vi "LineCrossed.vi"() -> (1 "LineDir":bool, 3 "Onside":bool)   [LabVIEW 2013]
uses:
  Robot Global Data.vi
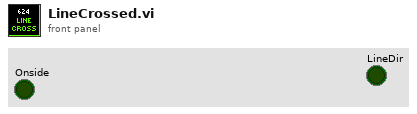
[diagram p1: front panel]
types:
  T1 = typedef "WPI_DriverStationAllianceInfo.ctl" = enum16{"Red", "Blue", "Invalid"}
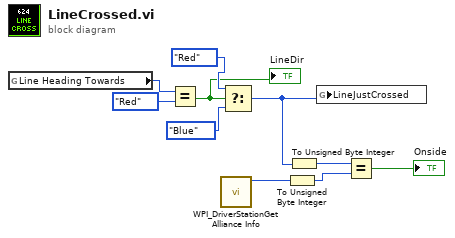
[diagram p0: block diagram]
diagram:
  n1 = global read "Robot Global Data.vi" "Line Heading Towards"() -> (w7:enum16{"Red", "Blue"})
  n2 = Equal?(x=w7, y=enum16{"Red", "Blue"}."Red") -> (x = y?=w5:bool)
  "LineDir" <- w5
  n3 = call <vilib>:"WPI_DriverStationGet Alliance Info.vi"() -> ("Alliance"=w4:T1)  [unwired: 10 in, 1 out]
  n4 = Select(t=enum16{"None", "Blue", "Red"}."Red" ("LineJustCrossed"), s=w5, f=enum16{"None", "Blue", "Red"}."Blue") -> (s? t:f=w2:enum16{"None", "Blue", "Red"})
  n5 = To Unsigned Byte Integer(number=w4) -> (unsigned 8bit integer=w3:u8)
  n6 = To Unsigned Byte Integer(number=w2) -> (unsigned 8bit integer=w1:u8)
  n7 = global write "Robot Global Data.vi" "LineJustCrossed"(w2) -> ()
  n8 = Equal?(x=w1, y=w3) -> (x = y?=→"Onside":bool)
